vi "xywav2x.vi"(3 "X or Y (X)":enum16{"X", "Y"}(ring), 4 "xywave":T1={"attributes"=variant, "Z"={"data"=[], "units"="au"}, "X"={"start"=0.0, "delta"=1.0, "units"="index", "dim"="x"}, "Y"={"start"=0.0, "delta"=1.0, "units"="index", "dim"="y"}}) -> (1 "X or Y (X)":dbl[](array[numeric]))   [LabVIEW 2015]
uses:
  xywav.ctl
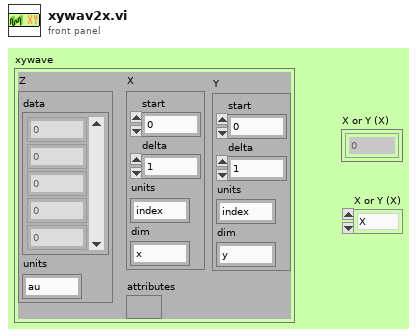
[diagram p1: front panel]
types:
  T1 = typedef "xywav.ctl" = cluster{"attributes":variant, "Z":cluster{"data":dbl[][], "units":string}, "X":cluster{"start":dbl, "delta":dbl, "units":string, "dim":string}, "Y":cluster{"start":dbl, "delta":dbl, "units":string, "dim":string}}
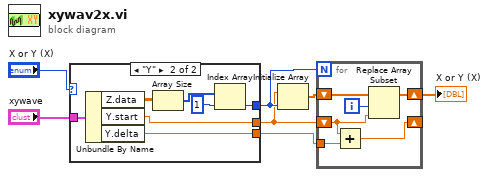
[diagram p0: block diagram]
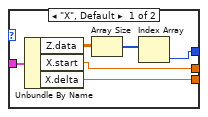
[diagram p2: hidden frame]
diagram:
  n1 = case shown="\"Y\"" "X or Y (X)" {
    tunnel: [w13 w19] -> w5
    tunnel: [w9 w15] -> w4
    tunnel: [w8 w14] -> w3
    tunnel: "xywave" -> [w11 w18]
    frame "X", Default {
      n2 = Unbundle By Name(w11) -> ("Z.data"=w10:dbl[][], "X.start"=w9:dbl, "X.delta"=w8:dbl)
      n3 = Array Size(array=w10) -> (size(s)=w12:i32[])
      n4 = Index Array(array=w12) -> (element=w13:i32)  [unwired: 1 in]
    }
    frame "Y" {
      n5 = Unbundle By Name(w18) -> ("Z.data"=w17:dbl[][], "Y.start"=w15:dbl, "Y.delta"=w14:dbl)
      n6 = Array Size(array=w17) -> (size(s)=w16:i32[])
      n7 = Index Array(array=w16, index=1) -> (element=w19:i32)
    }
  }
  n8 = Initialize Array(w4, w5) -> (w7:dbl[])
  n9 = for {
    N: w5 -> [_]
    shift-right: [w25] -> w6
    shift-left: w7 -> [w26]
    shift-right: [w21] -> _
    shift-left: w4 -> [w22]
    tunnel: w3 -> [w23]
    i -> [w24]
    n10 = Add(x=w22, y=w23) -> (x+y=w21:dbl)
    n11 = Replace Array Subset(array=w26, new element=w22, index=w24) -> (w25:dbl[])
  }
  "X or Y (X)" <- w6
